vi "OpenG Delete Elements from Array 1D Template.vi"(9 "indices":i32[](array[numeric]), 11 "array":dbl[](array[numeric]) format="%.2f") -> (1 "deleted elements":dbl[](array[numeric]) format="%.2f", 3 "array w/ subset deleted":dbl[](array[numeric]) format="%.2f")   [LabVIEW 2018]
doc: "This polymorphic VI deletes elements from a 1D or 2D <B>array</B> at the corresponding <B>indices</B>, returning <B>array w/ subset deleted</B> and <B>deleted elements</B>. For 2D arrays, wire the <B>delete (rows or columns)</B> input to specify whether to delete rows or columns."
panel:
  # "[OpenG VI Tags] ***Do Not Remove*** \nSVN Revision = 990\nSVN Revision Date = 2009-07-18 07:14:13 -0700 (Sat, 18 Jul 2009)\nPackage = oglib_array-3.0.0-1\nDepends ="
  # "Delete Elements from Array.vi\n\nThis polymorphic VI deletes elements from a 1D or 2D array at the corresponding indices\n\nPlease visit http://www.OpenG.org to learn about the\nOpen Source LabVIEW software movement.\n\nNOTICE -- YOU MUST LEAVE THIS NOTICE IN PLACE.  PER THE TERMS OF THE LICENSE BELOW, YOU MAY SUBLICENSE THIS SOFTWARE \nIN ANY WAY THAT DOES NOT CONFLICT WITH THIS LICENSE.\n\n### BSD License (http://www.opensource.org/licenses/bsd-license.php) Begin ###\n \nCopyright (c) 2007, JKI <info@jameskring.com> (Author: Jim Kring <jim.kring@jameskring.com>)\n\nAll rights reserved.\n\nRedistribution and use in source and binary forms, with or without modification, are permitted provided that the following conditions are met:\n\n    * Redistributions of source code must retain the above copyright notice, this list of conditions and the following disclaimer.\n    * Redistributions in binary form must reproduce the above copyright notice, this list of conditions and the following disclaimer in the \n       documentation and/or other materials provided with the distribution.\n    * Neither the name of SciWare, James Kring, Inc., nor the names of its contributors may be used to endorse or promote products derived \n       from this software without specific prior written permission.\n\nTHIS SOFTWARE IS PROVIDED BY THE COPYRIGHT HOLDERS AND CONTRIBUTORS \"AS IS\" AND ANY EXPRESS OR IMPLIED WARRANTIES, \nINCLUDING, BUT NOT LIMITED TO, THE IMPLIED WARRANTIES OF MERCHANTABILITY AND FITNESS FOR A PARTICULAR PURPOSE ARE \nDISCLAIMED. IN NO EVENT SHALL THE COPYRIGHT OWNER OR CONTRIBUTORS BE LIABLE FOR ANY DIRECT, INDIRECT, INCIDENTAL,\n SPECIAL, EXEMPLARY, OR CONSEQUENTIAL DAMAGES (INCLUDING, BUT NOT LIMITED TO, PROCUREMENT OF SUBSTITUTE GOODS OR \nSERVICES; LOSS OF USE, DATA, OR PROFITS; OR BUSINESS INTERRUPTION) HOWEVER CAUSED AND ON ANY THEORY OF LIABILITY, \nWHETHER IN CONTRACT, STRICT LIABILITY, OR TORT (INCLUDING NEGLIGENCE OR OTHERWISE) ARISING IN ANY WAY OUT OF THE USE \nOF THIS SOFTWARE, EVEN IF ADVISED OF THE POSSIBILITY OF SUCH DAMAGE.\n\n### BSD License End ###"
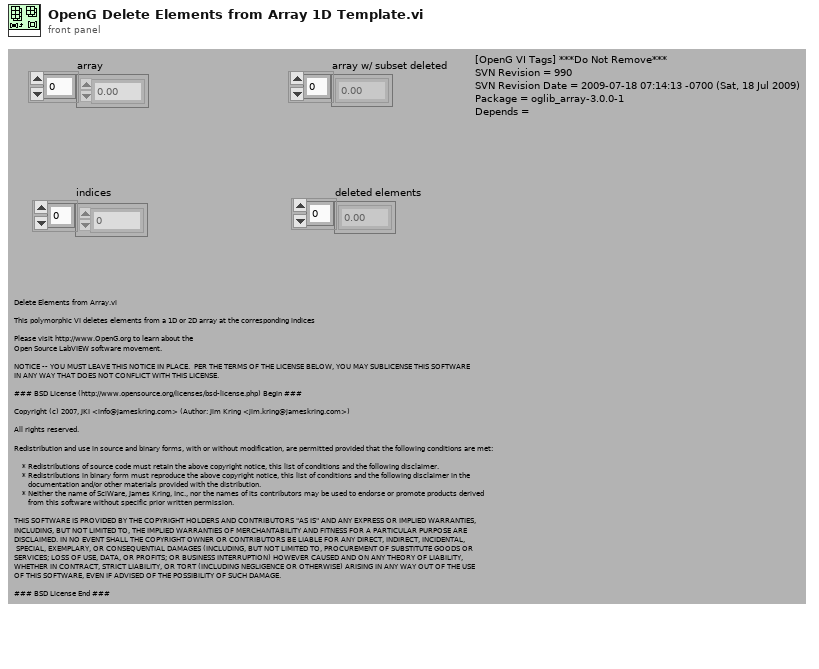
[diagram p1: front panel]
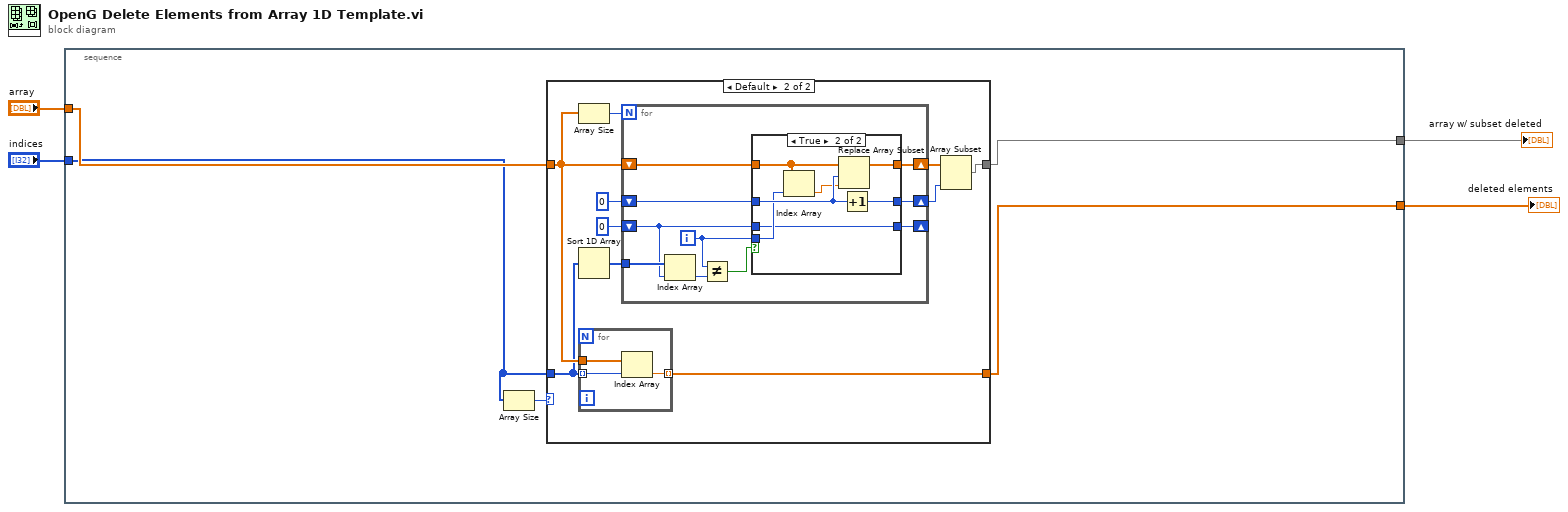
[diagram p0: block diagram]
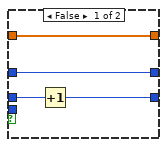
[diagram p3: hidden frame]
diagram:
  n1 = stacked-sequence {
    tunnel: "array" -> [w8]
    tunnel: [w6] -> w3
    tunnel: "indices" -> [w7]
    tunnel: [w5] -> w1
    frame #0 {
      n2 = Array Size(array=w7) -> (size(s)=w9:i32)
      n3 = case shown="Default" w9 {
        tunnel: [w10 w15] -> w6
        tunnel: w8 -> [w10 w14]
        tunnel: [_ w13] -> w5
        tunnel: w7 -> [_ w12]
        frame 0 {
        }
        frame Default {
          n4 = Array Size(array=w14) -> (size(s)=w20:i32)
          n5 = Sort 1D Array(array=w12) -> (sorted array=w11:i32[])
          n6 = for {
            tunnel: w12 -> [w22] mode=indexing
            tunnel: w14 -> [w23]
            tunnel: [w21] -> w13 mode=indexing
            n7 = Index Array(array=w23, index=w22) -> (element=w21:dbl)
          }
          n8 = for {
            N: w20 -> [_]
            shift-right: [w28] -> w16
            shift-left: w14 -> [w32]
            shift-right: [w30] -> w17
            shift-left: 0 -> [w31]
            shift-right: [w24] -> _
            shift-left: 0 -> [w25]
            tunnel: w11 -> [w27]
            i -> [w29]
            n9 = Index Array(array=w27, index=w25) -> (element=w26:i32)
            n10 = Not Equal?(x=w29, y=w26) -> (x != y?=w33:bool)
            n11 = case shown="True" w33 {
              tunnel: w32 -> [w36 w38]
              tunnel: w31 -> [w37 w43]
              tunnel: [w37 w44] -> w30
              tunnel: w29 -> [_ w42]
              tunnel: [w36 w40] -> w28
              tunnel: w25 -> [w35 w39]
              tunnel: [w34 w39] -> w24
              frame False {
                n12 = Increment(x=w35) -> (x+1=w34:i32)
              }
              frame True {
                n13 = Index Array(array=w38, index=w42) -> (element=w41:dbl)
                n14 = Replace Array Subset(array=w38, new element=w41, index=w43) -> (w40:dbl[])
                n15 = Increment(x=w43) -> (x+1=w44:i32)
              }
            }
          }
          n16 = Array Subset(array=w16, length=w17) -> (w15:dbl[])  [unwired: 1 in]
        }
      }
    }
  }
  "array w/ subset deleted" <- w3
  "deleted elements" <- w1
